vi "FPGA_R_ADC_W_DAC.vi"() -> ()   [LabVIEW 2019]
uses:
  <vilib>/rvi/Emulation/niFpgaGetClockAttributes.vi
  <vilib>/rvi/Emulation/niFpgaSctlEmulationGetInTimedLoop.vi
  <vilib>/rvi/Emulation/niFpgaEmulationReportErrorSimple.vi
  <vilib>/rvi/eio/common/nirviEmuTemplateMethod_errors.vi
  <vilib>/rvi/Emulation/niFpgaCriticalErrorInLSC.vi
  <vilib>/eio/EIONode/EIONode.xnode
panel:
  in  "stop 3":bool
  out "Data array 3":bool[](array[boolean])
  in  "stop 2":bool
  out "Data array 2":bool[](array[boolean])
  out "Encoder B Ref":bool
  out "Encoder A Ref":bool
  out "Encoder B":i32
  out "Encoder A":i32
  in  "ENC stop":bool
  in  "Count(Ticks)":u32=800
  in  "DAC 3 write":bool[](array[boolean])=[FALSE, FALSE, FALSE, FALSE, FALSE, FALSE, FALSE, FALSE, FALSE, FALSE, FALSE, FALSE, FALSE, FALSE, FALSE, FALSE]
  in  "DAC 2 write":bool[](array[boolean])=[FALSE, FALSE, FALSE, FALSE, FALSE, FALSE, FALSE, FALSE, FALSE, FALSE, FALSE, FALSE, FALSE, FALSE, FALSE, FALSE]
  in  "DAC 1 write":bool[](array[boolean])=[FALSE, FALSE, FALSE, FALSE, FALSE, FALSE, FALSE, FALSE, FALSE, FALSE, FALSE, FALSE, FALSE, FALSE, FALSE, FALSE]
  out "ADC read":bool[](array[boolean])
  in  "ADC write":bool[](array[boolean])=[FALSE, FALSE, FALSE, FALSE, FALSE, TRUE, FALSE, FALSE, FALSE, FALSE, FALSE, FALSE, FALSE, FALSE, FALSE, FALSE]
  in  "DAQ stop":bool
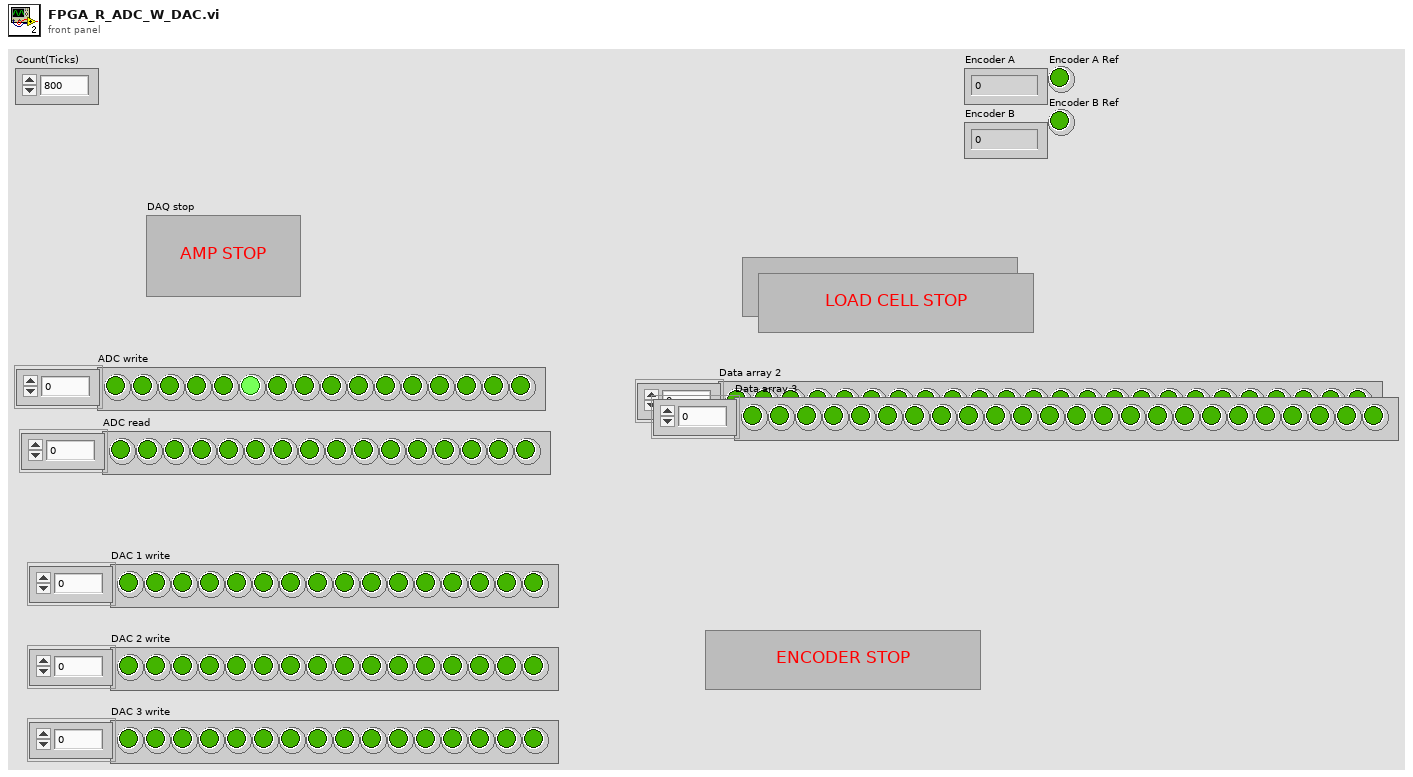
[diagram p1: front panel]
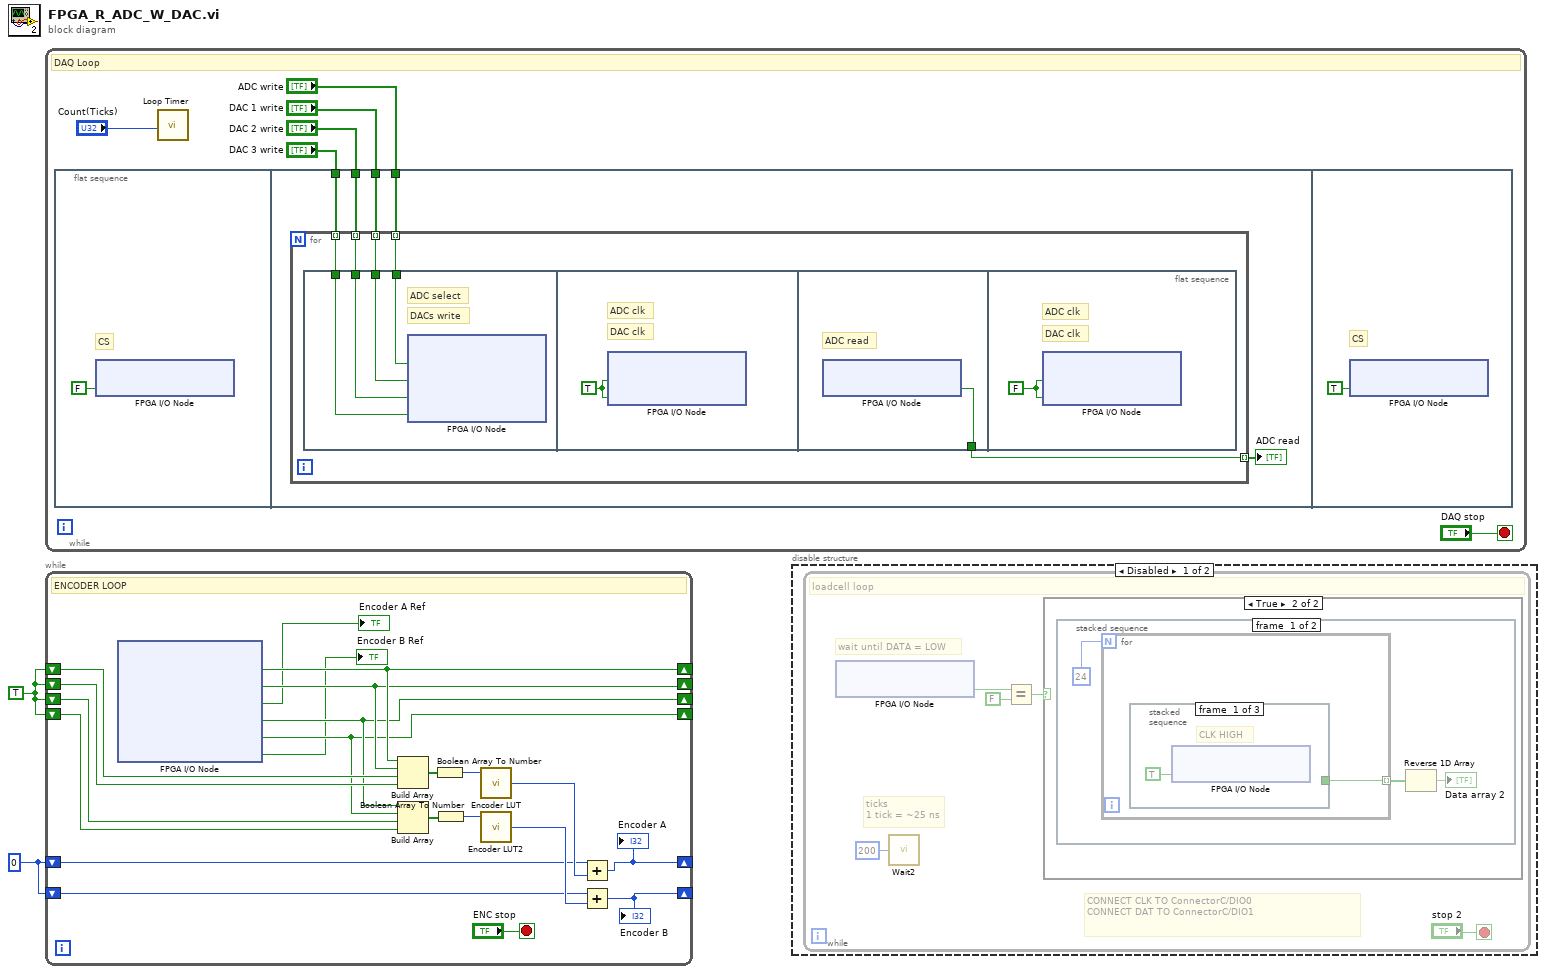
[diagram p0: block diagram]
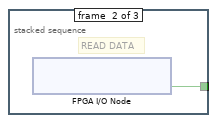
[diagram p3: hidden frame]
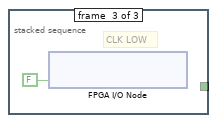
[diagram p4: hidden frame]
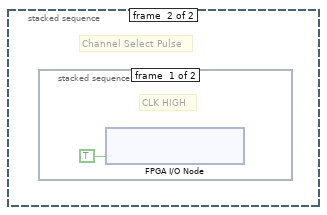
[diagram p5: hidden frame]
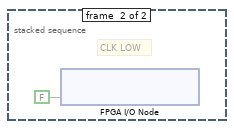
[diagram p6: hidden frame]
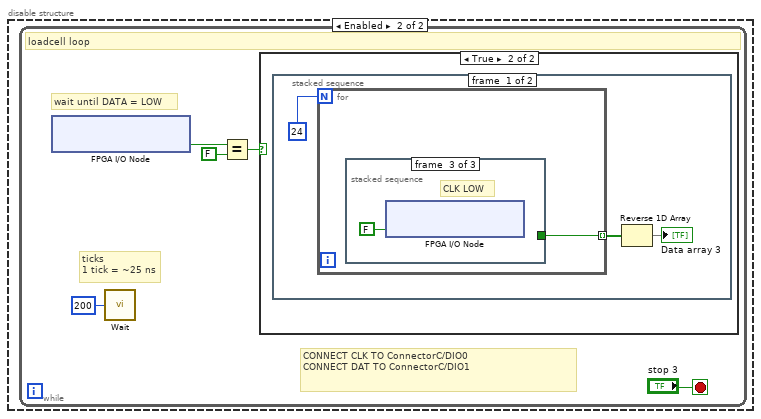
[diagram p7: hidden frame]
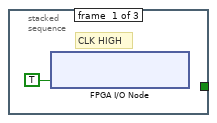
[diagram p9: hidden frame]
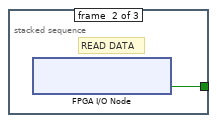
[diagram p10: hidden frame]
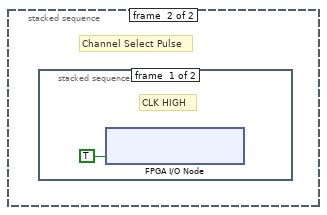
[diagram p11: hidden frame]
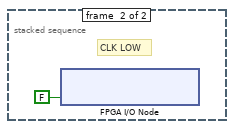
[diagram p12: hidden frame]
diagram:
  w1 = TRUE
  w2 = 0
  n1 = while {
    stop <- "DAQ stop" stop-if-true
    # "DAQ Loop"
    n2 = flat-sequence {
      tunnel: "ADC write" -> [w14]
      tunnel: "DAC 1 write" -> [w13]
      tunnel: "DAC 2 write" -> [w12]
      tunnel: "DAC 3 write" -> [w11]
      frame #0 {
        # "CS"
        n3 = xnode "FPGA I/O Node"("ConnectorA/DIO4"=FALSE) -> ()  [unwired: 1 in, 1 out]
      }
      frame #1 {
        n4 = for {
          tunnel: w14 -> [w19] mode=indexing
          tunnel: w13 -> [w18] mode=indexing
          tunnel: w12 -> [w17] mode=indexing
          tunnel: w11 -> [w16] mode=indexing
          tunnel: [w15] -> w10 mode=indexing
          n5 = flat-sequence {
            tunnel: w19 -> [w23]
            tunnel: w18 -> [w20]
            tunnel: w17 -> [w22]
            tunnel: w16 -> [w21]
            tunnel: [w25] -> w15
            frame #0 {
              # "DACs write"
              # "ADC select"
              n6 = xnode "FPGA I/O Node"("ConnectorA/DIO2"=w23, "ConnectorA/DIO6"=w20, "ConnectorA/DIO7"=w22, "ConnectorA/DIO8"=w21) -> ()  [unwired: 4 in, 4 out]
            }
            frame #1 {
              w24 = TRUE ("ConnectorA/DIO3")
              # "DAC clk"
              # "ADC clk"
              n7 = xnode "FPGA I/O Node"("ConnectorA/DIO3"=w24, "ConnectorA/DIO5"=w24) -> ()  [unwired: 2 in, 2 out]
            }
            frame #2 {
              # "ADC read"
              n8 = xnode "FPGA I/O Node"() -> ("ConnectorA/DIO1"=w25:bool)  [unwired: 1 in, 1 out]
            }
            frame #3 {
              w26 = FALSE ("ConnectorA/DIO3")
              # "DAC clk"
              # "ADC clk"
              n9 = xnode "FPGA I/O Node"("ConnectorA/DIO3"=w26, "ConnectorA/DIO5"=w26) -> ()  [unwired: 2 in, 2 out]
            }
          }
        }
        "ADC read" <- w10
      }
      frame #2 {
        # "CS"
        n10 = xnode "FPGA I/O Node"("ConnectorA/DIO4"=TRUE) -> ()  [unwired: 1 in, 1 out]
      }
    }
    n11 = call "Loop Timer"("Count(Ticks)"="Count(Ticks)") -> ()  [unwired: 1 out]
  }
  n12 = while {
    shift-right: [w29] -> _
    shift-left: w2 -> [w32]
    shift-right: [w37] -> _
    shift-left: w1 -> [w47]
    shift-right: [w36] -> _
    shift-left: w1 -> [w42]
    shift-right: [w35] -> _
    shift-left: w1 -> [w41]
    shift-right: [w34] -> _
    shift-left: w1 -> [w40]
    shift-right: [w30] -> _
    shift-left: w2 -> [w31]
    stop <- "ENC stop" stop-if-true
    # "ENCODER LOOP"
    n13 = xnode "FPGA I/O Node"() -> ("ConnectorA/DIO9"=w37:bool, "ConnectorA/DIO10"=w36:bool, "ConnectorA/DIO11"=→"Encoder A Ref":bool, "ConnectorA/DIO13"=w35:bool, "ConnectorA/DIO14"=w34:bool, "ConnectorA/DIO12"=→"Encoder B Ref":bool)  [unwired: 6 in, 6 out]
    n14 = Build Array(w37, w36, w47, w42) -> (w45:bool[])
    n15 = Build Array(w35, w34, w41, w40) -> (w46:bool[])
    n16 = Boolean Array To Number(Boolean array=w45) -> (number=w44:u8)
    n17 = Boolean Array To Number(Boolean array=w46) -> (number=w43:u8)
    n18 = call "Encoder LUT"("address"=w44) -> ("data out"=w39:i32)  [unwired: 8 in]
    n19 = call "Encoder LUT2"("address"=w43) -> ("data out"=w38:i32)  [unwired: 8 in]
    n20 = Add(x=w32, y=w39) -> (x+y=w29:i32)
    "Encoder A" <- w29
    n21 = Add(x=w31, y=w38) -> (x+y=w30:i32)
    "Encoder B" <- w30
  }
  n22 = disable-structure shown="Disabled" {
    frame Disabled {
      n23 = while {
        stop <- "stop 2" stop-if-true
        # "CONNECT CLK TO ConnectorC/DIO0\nCONNECT DAT TO ConnectorC/DIO1"
        # "ticks\n1 tick = ~25 ns"
        # "wait until DATA = LOW"
        # "loadcell loop"
        n24 = xnode "FPGA I/O Node"() -> ("ConnectorC/DIO1"=w52:bool)  [unwired: 1 in, 1 out]
        n25 = call "Wait2"("Count(Ticks)"=u32 200) -> ()  [unwired: 1 out]
        n26 = Equal?(x=w52, y=FALSE) -> (x = y?=w50:bool)
        n27 = case shown="True" w50 {
          frame False {
          }
          frame True {
            n28 = stacked-sequence {
              frame #0 {
                n29 = for {
                  N: 24 -> [_]
                  tunnel: [w57] -> w55 mode=indexing
                  n30 = stacked-sequence {
                    tunnel: [_ w59 _] -> w57
                    frame #0 {
                      # "CLK HIGH"
                      n31 = xnode "FPGA I/O Node"("ConnectorC/DIO0"=TRUE ("ConnectorB/DIO0")) -> ()  [unwired: 1 in, 1 out]
                    }
                    frame #1 {
                      # "READ DATA"
                      n32 = xnode "FPGA I/O Node"() -> ("ConnectorC/DIO1"=w59:bool)  [unwired: 1 in, 1 out]
                    }
                    frame #2 {
                      # "CLK LOW"
                      n33 = xnode "FPGA I/O Node"("ConnectorC/DIO0"=FALSE ("ConnectorB/DIO0")) -> ()  [unwired: 1 in, 1 out]
                    }
                  }
                }
                n34 = Reverse 1D Array(array=w55) -> (reversed array=→"Data array 2":bool[])
              }
              frame #1 {
                # "Channel Select Pulse"
                n35 = stacked-sequence {
                  frame #0 {
                    # "CLK HIGH"
                    n36 = xnode "FPGA I/O Node"("ConnectorC/DIO0"=TRUE ("ConnectorB/DIO0")) -> ()  [unwired: 1 in, 1 out]
                  }
                  frame #1 {
                    # "CLK LOW"
                    n37 = xnode "FPGA I/O Node"("ConnectorC/DIO0"=FALSE ("ConnectorB/DIO0")) -> ()  [unwired: 1 in, 1 out]
                  }
                }
              }
            }
          }
        }
      }
    }
    frame Enabled {
      n38 = while {
        stop <- "stop 3" stop-if-true
        # "CONNECT CLK TO ConnectorC/DIO0\nCONNECT DAT TO ConnectorC/DIO1"
        # "ticks\n1 tick = ~25 ns"
        # "wait until DATA = LOW"
        # "loadcell loop"
        n39 = xnode "FPGA I/O Node"() -> ("ConnectorC/DIO1"=w66:bool)  [unwired: 1 in, 1 out]
        n40 = call "Wait"("Count(Ticks)"=u32 200) -> ()  [unwired: 1 out]
        n41 = Equal?(x=w66, y=FALSE) -> (x = y?=w64:bool)
        n42 = case shown="True" w64 {
          frame False {
          }
          frame True {
            n43 = stacked-sequence {
              frame #0 {
                n44 = for {
                  N: 24 -> [_]
                  tunnel: [w71] -> w69 mode=indexing
                  n45 = stacked-sequence {
                    tunnel: [_ w73 _] -> w71
                    frame #0 {
                      # "CLK HIGH"
                      n46 = xnode "FPGA I/O Node"("ConnectorC/DIO0"=TRUE ("ConnectorB/DIO0")) -> ()  [unwired: 1 in, 1 out]
                    }
                    frame #1 {
                      # "READ DATA"
                      n47 = xnode "FPGA I/O Node"() -> ("ConnectorC/DIO1"=w73:bool)  [unwired: 1 in, 1 out]
                    }
                    frame #2 {
                      # "CLK LOW"
                      n48 = xnode "FPGA I/O Node"("ConnectorC/DIO0"=FALSE ("ConnectorB/DIO0")) -> ()  [unwired: 1 in, 1 out]
                    }
                  }
                }
                n49 = Reverse 1D Array(array=w69) -> (reversed array=→"Data array 3":bool[])
              }
              frame #1 {
                # "Channel Select Pulse"
                n50 = stacked-sequence {
                  frame #0 {
                    # "CLK HIGH"
                    n51 = xnode "FPGA I/O Node"("ConnectorC/DIO0"=TRUE ("ConnectorB/DIO0")) -> ()  [unwired: 1 in, 1 out]
                  }
                  frame #1 {
                    # "CLK LOW"
                    n52 = xnode "FPGA I/O Node"("ConnectorC/DIO0"=FALSE ("ConnectorB/DIO0")) -> ()  [unwired: 1 in, 1 out]
                  }
                }
              }
            }
          }
        }
      }
    }
  }
